vi "LeerBD.vi"(8 "error in (no error)":errorcluster) -> (0 "error out":errorcluster, 1 "clase":i32, 2 "BD":T1)   [LabVIEW 2019, in "Prueba21.lvclass"]
uses:
  Prueba21.lvclass
  BD.ctl
  Base de Datos/SQLiteConnector/SQLiteConnection.lvclass
  Base de Datos/Base de Datos.lvclass
panel:
  in  "Tipo Equipo":enum16{"Sonometro", "Calibrador", "Dosimetro"}(ring)
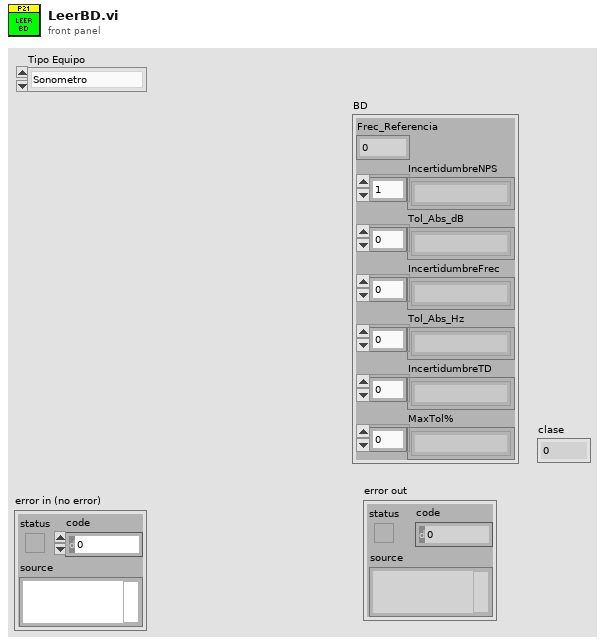
[diagram p1: front panel]
types:
  T1 = typedef "Prueba21.lvclass/BD.ctl" = cluster{"Frec_Referencia":dbl, "IncertidumbreNPS":string[], "Tol_Abs_dB":string[], "IncertidumbreFrec":string[], "Tol_Abs_Hz":string[], "IncertidumbreTD":string[], "MaxTol%":string[]}
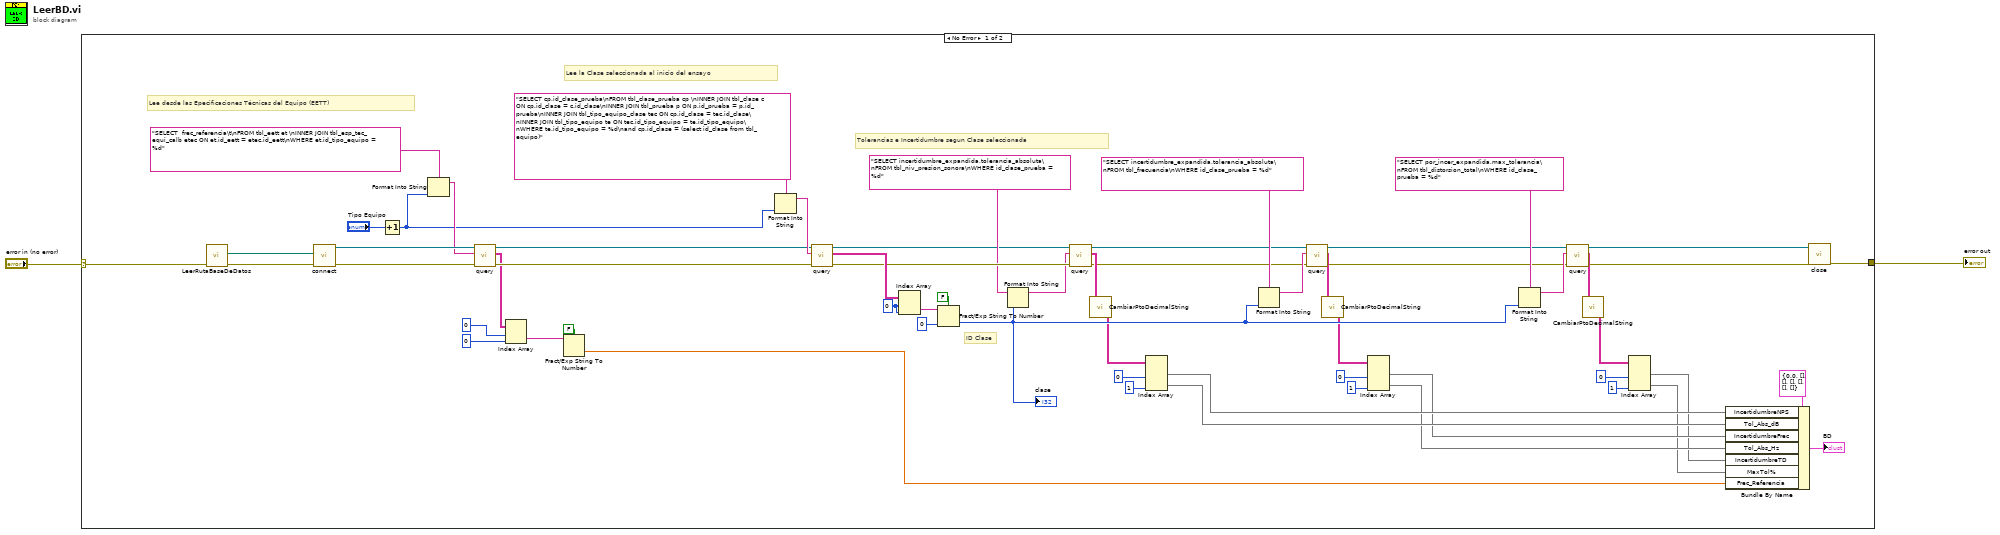
[diagram p0: block diagram]
diagram:
  n1 = case shown="No Error" "error in (no error)" {
    selector: "error in (no error)" -> [w55 w63]
    tunnel: [w41 w63] -> w1
    frame No Error {
      w47 = 0 ("index (row)")
      # "Tolerancias e Incertidumbre segun Clase seleccionada"
      # "ID Clase"
      # "Lee la Clase seleccionada al inicio del ensayo"
      # "Lee desde las Epecificaciones Técnicas del Equipo (EETT)"
      n2 = call "LeerRutaBaseDeDatos.vi"("error in (no error)"=w55) -> ("error out"=w58:errorcluster, "Database Path"=w57:path)  [unwired: 9 in]
      n3 = call "connect.vi"("error in (no error)"=w58, "Database Path"=w57) -> ("error out"=w60:errorcluster, "object out"=w61:refnum<class "SQLiteConnection.lvclass">)  [unwired: 8 in]
      n4 = Increment(x="Tipo Equipo") -> (x+1=w37:enum16{"Sonometro", "Calibrador", "Dosimetro"})
      n5 = Format Into String(format string="SELECT  frec_referencia\t\nFROM tbl_eett et \nINNER JOIN tbl_esp_tec_equi_calb etec ON et.id_eett = etec.id_eett\nWHERE et.id_tipo_equipo = %d", w37) -> (resulting string=w59:string)  [unwired: 2 in, 1 out]
      n6 = call "query.vi"("error in (no error)"=w60, "SQL Statement"=w59, "object in"=w61) -> ("error out"=w48:errorcluster, "result"=w33:string[][], "object out"=w49:refnum<class "SQLiteConnection.lvclass">)  [unwired: 5 in, 1 out]
      n7 = Index Array(array=w33, index (row)=0, index (col)=0 ("disabled index (col)")) -> (element=w53:string)
      n8 = Fract/Exp String To Number(use system decimal point (T)=FALSE, string=w53) -> (number=w12:dbl)  [unwired: 2 in, 1 out]
      n9 = Format Into String(format string="SELECT cp.id_clase_prueba\nFROM tbl_clase_prueba cp \nINNER JOIN tbl_clase c ON cp.id_clase = c.id_clase\nINNER JOIN tbl_prueba p ON p.id_prueba = p.id_prueba\nINNER JOIN tbl_tipo_equipo_clase tec ON cp.id_clase = tec.id_clase\nINNER JOIN tbl_tipo_equipo te ON tec.id_tipo_equipo = te.id_tipo_equipo\nWHERE te.id_tipo_equipo = %d\nand cp.id_clase = (select id_clase from tbl_equipo)", w37) -> (resulting string=w50:string)  [unwired: 2 in, 1 out]
      n10 = call "query.vi"("error in (no error)"=w48, "SQL Statement"=w50, "object in"=w49) -> ("error out"=w42:errorcluster, "result"=w43:string[][], "object out"=w39:refnum<class "SQLiteConnection.lvclass">)  [unwired: 5 in, 1 out]
      n11 = Index Array(array=w43, index (row)=w47, index (col)=w47) -> (element=w45:string)
      n12 = Fract/Exp String To Number(use system decimal point (T)=FALSE, string=w45, default (0 dbl)=0 ("index (row)")) -> (number=w21:i32)  [unwired: 1 in, 1 out]
      "clase" <- w21
      n13 = Format Into String(format string="SELECT incertidumbre_expandida,tolerancia_absoluta\nFROM tbl_niv_presion_sonora\nWHERE id_clase_prueba = %d", w21) -> (resulting string=w38:string)  [unwired: 2 in, 1 out]
      n14 = call "query.vi"("error in (no error)"=w42, "SQL Statement"=w38, "object in"=w39) -> ("error out"=w8:errorcluster, "result"=w36:string[][], "object out"=w11:refnum<class "SQLiteConnection.lvclass">)  [unwired: 5 in, 1 out]
      n15 = call "CambiarPtoDecimalString.vi"("result"=w36) -> ("result out"=w3:string[][])
      n16 = Index Array(array=w3, index (col) #1=0 ("disabled index (col)"), index (col) #2=1 ("disabled index (col)")) -> (element #1=w31:string[], element #2=w30:string[])  [unwired: 2 in]
      n17 = Format Into String(format string="SELECT incertidumbre_expandida,tolerancia_absoluta\nFROM tbl_frecuencia\nWHERE id_clase_prueba = %d", w21) -> (resulting string=w19:string)  [unwired: 2 in, 1 out]
      n18 = call "query.vi"("error in (no error)"=w8, "SQL Statement"=w19, "object in"=w11) -> ("error out"=w7:errorcluster, "result"=w18:string[][], "object out"=w10:refnum<class "SQLiteConnection.lvclass">)  [unwired: 5 in, 1 out]
      n19 = call "CambiarPtoDecimalString.vi"("result"=w18) -> ("result out"=w4:string[][])
      n20 = Index Array(array=w4, index (col) #1=0 ("disabled index (col)"), index (col) #2=1 ("disabled index (col)")) -> (element #1=w16:string[], element #2=w15:string[])  [unwired: 2 in]
      n21 = Format Into String(format string="SELECT por_incer_expandida,max_tolerancia\nFROM tbl_distorsion_total\nWHERE id_clase_prueba = %d", w21) -> (resulting string=w20:string)  [unwired: 2 in, 1 out]
      n22 = call "query.vi"("error in (no error)"=w7, "SQL Statement"=w20, "object in"=w10) -> ("error out"=w6:errorcluster, "result"=w17:string[][], "object out"=w9:refnum<class "SQLiteConnection.lvclass">)  [unwired: 5 in, 1 out]
      n23 = call "CambiarPtoDecimalString.vi"("result"=w17) -> ("result out"=w5:string[][])
      n24 = Index Array(array=w5, index (col) #1=0 ("disabled index (col)"), index (col) #2=1 ("disabled index (col)")) -> (element #1=w14:string[], element #2=w13:string[])  [unwired: 2 in]
      n25 = Bundle By Name(cluster=T1 {"Frec_Referencia"=0.0, "IncertidumbreNPS"=[], "Tol_Abs_dB"=[], "IncertidumbreFrec"=[], "Tol_Abs_Hz"=[], "IncertidumbreTD"=[], "MaxTol%"=[]} ("BD"), "IncertidumbreNPS"=w31, "Tol_Abs_dB"=w30, "IncertidumbreFrec"=w16, "Tol_Abs_Hz"=w15, "IncertidumbreTD"=w14, "MaxTol%"=w13, "Frec_Referencia"=w12) -> (→"BD":T1)
      n26 = call-dynamic "close.vi"("error in (no error)"=w6, "object in"=w9) -> ("error out"=w41:errorcluster)  [unwired: 8 in, 1 out]
    }
    frame Error {
    }
  }
  "error out" <- w1
